vi "circle plots.vi"() -> ()   [LabVIEW 2017]
doc: "Developed by Kevin Thompson\nkevin@thompsonengineering.net\n\nCopyright 2018-2020\nThompson Engineering, LLC"
uses:
  <userlib>/_OpenG.lib/numeric/numeric.llb/Random Number Within Range - DBL__ogtk.vi
panel:
  in  "stop":bool
  out "XY Graph":cluster{dbl[], dbl[]}[](graph)=[{[9.998476951563912], [-0.1745240643728356]}, {array[360 elements], array[360 elements]}, {array[360 elements], array[360 elements]}, {array[360 elements], array[360 elements]}]
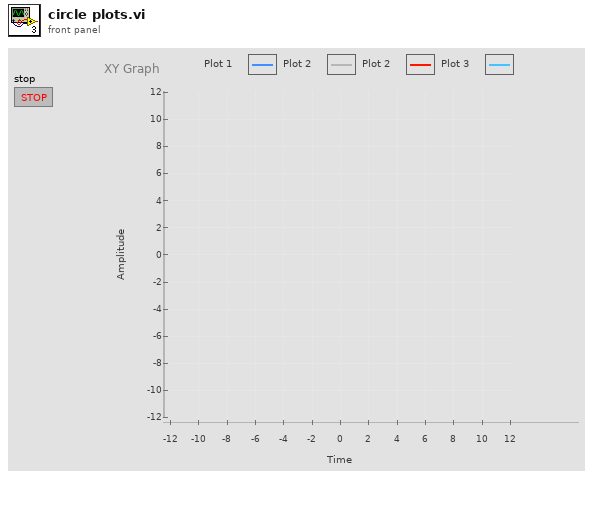
[diagram p1: front panel]
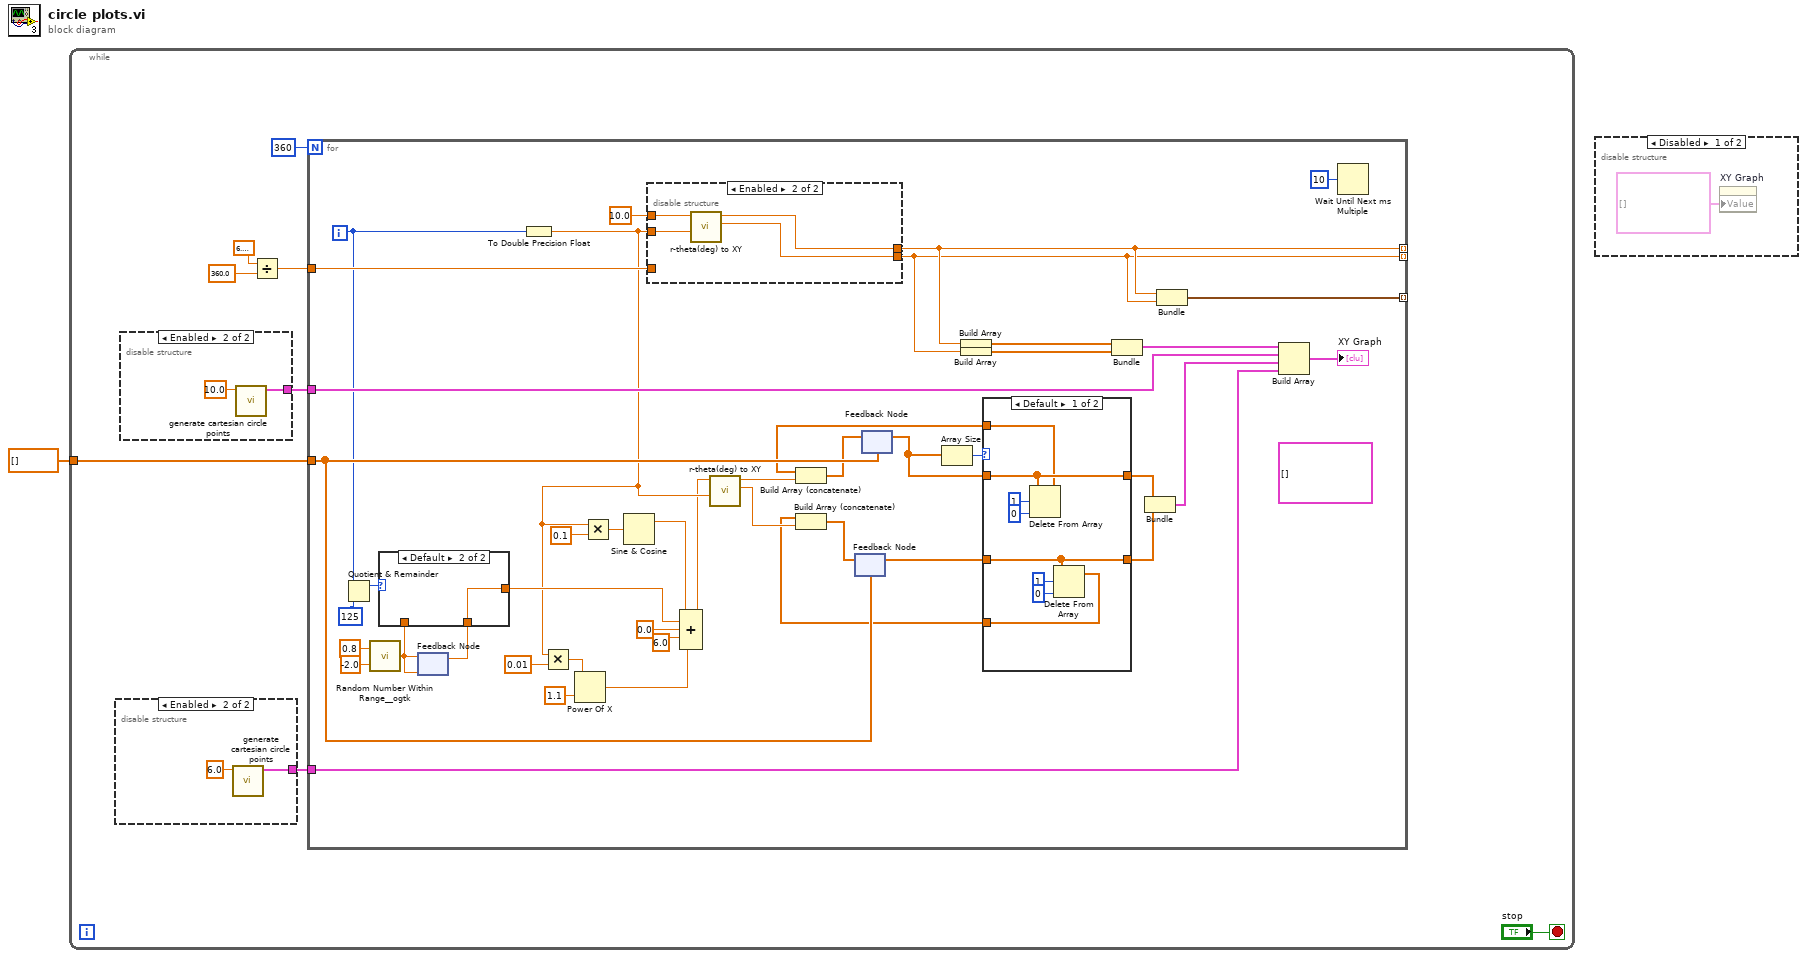
[diagram p0: block diagram]
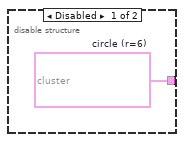
[diagram p3: hidden frame]
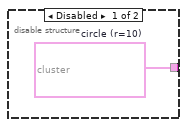
[diagram p4: hidden frame]
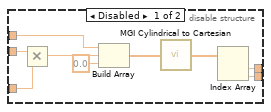
[diagram p7: hidden frame]
diagram:
  n1 = while {
    tunnel: dbl[] [] -> [w2]
    stop <- "stop" stop-if-true
    n2 = disable-structure shown="Enabled" {
      disable-tunnel: [w10 w11] -> w4
      frame Disabled {
        w10 = cluster{dbl[], dbl[]} {array[360 elements], array[360 elements]}  # circle (r=6)
      }
      frame Enabled {
        n3 = call "generate cartesian circle points.vi"("radius (deg)"=6.0) -> ("circle XY"=w11:cluster{"X[]":dbl[], "Y[]":dbl[]})  [unwired: 10 in]
      }
    }
    n4 = disable-structure shown="Enabled" {
      disable-tunnel: [w13 w14] -> w5
      frame Disabled {
        w13 = cluster{dbl[], dbl[]} {array[360 elements], array[360 elements]}  # circle (r=10)
      }
      frame Enabled {
        n5 = call "generate cartesian circle points.vi"("radius (deg)"=10.0) -> ("circle XY"=w14:cluster{"X[]":dbl[], "Y[]":dbl[]})  [unwired: 10 in]
      }
    }
    n6 = Divide(x=6.283185307179586, y=360.0) -> (x/y=w6:dbl)
    n7 = for {
      N: 360 -> [_]
      tunnel: w5 -> [w53]
      tunnel: [w52] -> _ mode=indexing
      tunnel: [w51] -> _ mode=indexing
      tunnel: w6 -> [w55]
      tunnel: [w50] -> _ mode=indexing
      tunnel: w4 -> [w49]
      tunnel: w2 -> [w45]
      i -> [w26]
      (unwired) cluster{"X[]":dbl[], "Y[]":dbl[]}[] [] ("appended array")
      n8 = Quotient & Remainder(x=w26, y=125) -> (x-y*floor(x/y)=w27:i32)  [unwired: 1 out]
      n9 = call-poly <userlib>:"Random Number Within Range__ogtk.vi"("High"=0.8, "Low"=-2.0) -> ("Random Number"=w22:dbl)  [unwired: 3 in]
      n10 = feedback #1(w22) -> (w21:dbl)
      n11 = case shown="Default" w27 {
        tunnel: w22 -> [w60 _]
        tunnel: w21 -> [_ w61]
        tunnel: [w60 w61] -> w19
        frame 0 {
        }
        frame Default {
        }
      }
      n12 = feedback-in #1(w22) -> ()
      n13 = To Double Precision Float(number=w26) -> (double precision float=w17:dbl)
      n14 = Multiply(x=w17, y=0.01) -> (x*y=w30:dbl)
      n15 = Power Of X(1:1.1 ("x"), 2:w30) -> (0:w29:dbl)
      n16 = Multiply(x=w17, y=0.1) -> (x*y=w36:dbl)
      n17 = Sine & Cosine(0:w36) -> (1:w20:dbl)  [unwired: 1 out]
      n18 = disable-structure shown="Enabled" {
        disable-tunnel: w17 -> [w77 w82]
        disable-tunnel: w55 -> [w76 _]
        disable-tunnel: [w74 w84] -> w52
        disable-tunnel: [w73 w83] -> w51
        disable-tunnel: 10.0 ("circle radius") -> [w72 w81]
        frame Disabled {
          n19 = Multiply(x=w77, y=w76) -> (x*y=w75:dbl)
          n20 = Build Array(w72, w75, 0.0 ("element")) -> (w79:dbl[])
          n21 = call <userlib>:"MGI Cylindrical to Cartesian.vi"("R,Th,Z"=w79) -> ("X,Y,Z"=w78:dbl[])
          n22 = Index Array(array=w78) -> (element #1=w74:dbl, element #2=w73:dbl)  [unwired: 2 in]
        }
        frame Enabled {
          n23 = call "r-theta(deg) to XY.vi"("deg [0,360]"=w82, "circle radius"=w81) -> ("Y"=w83:dbl, "X"=w84:dbl)  [unwired: 6 in, 2 out]
        }
      }
      n24 = Compound Arithmetic op=ADD(w20, w19, 0.0 ("value"), 6.0 ("circle radius"), w29) -> (w16:dbl)
      n25 = call "r-theta(deg) to XY.vi"("deg [0,360]"=w17, "circle radius"=w16) -> ("Y"=w47:dbl, "X"=w48:dbl)  [unwired: 6 in, 2 out]
      n26 = feedback #2(w45) -> (w40:dbl[])
      n27 = feedback #3(w45) -> (w41:dbl[])
      n28 = Array Size(array=w41) -> (size(s)=w44:i32)
      n29 = Build Array(w52) -> (w59:dbl[])
      n30 = Build Array(w51) -> (w58:dbl[])
      n31 = case shown="Default" w44 {
        tunnel: w41 -> [w69 w70]
        tunnel: [w69 w70] -> w42
        tunnel: w40 -> [w63 w71]
        tunnel: [w63 w71] -> w39
        tunnel: [w62 w71] -> w28
        tunnel: [w68 w70] -> w37
        frame Default {
          n32 = Delete From Array(array=w69, length=1, index=0) -> (array with subset deleted=w68:dbl[])  [unwired: 1 out]
          n33 = Delete From Array(array=w63, length=1, index=0) -> (array with subset deleted=w62:dbl[])  [unwired: 1 out]
        }
        frame 0..359 {
        }
      }
      n34 = Build Array (concatenate)(w37, w48) -> (w43:dbl[])
      n35 = Build Array (concatenate)(w28, w47) -> (w38:dbl[])
      n36 = feedback-in #2(w38) -> ()
      n37 = feedback-in #3(w43) -> ()
      n38 = Bundle(w59, w58) -> (w54:cluster{dbl[], dbl[]})  [unwired: 1 in]
      n39 = Bundle(w42, w39) -> (w46:cluster{dbl[], dbl[]})  [unwired: 1 in]
      n40 = Bundle("X"=w52, "Y"=w51) -> (w50:cluster{"X":dbl, "Y":dbl})  [unwired: 1 in]
      n41 = Build Array(w54, w53, w46, w49) -> (→"XY Graph":cluster{"X[]":dbl[], "Y[]":dbl[]}[])
      n42 = Wait Until Next ms Multiple(millisecond multiple=u32 10) -> ()  [unwired: 1 out]
    }
  }
  n43 = disable-structure shown="Disabled" {
    frame Disabled {
      n44 = property on="XY Graph" class="XYGraph (strict)"("Value"=cluster{dbl[], dbl[]}[] [] ("XY Graph")) -> ()  [unwired: 2 in, 2 out]
    }
    frame Enabled {
    }
  }
